vi "CSM - Check Status Registration.vi"(8 "error in (no error)":errorcluster, 10 "CSM Name":string, 11 "Broadcast state":string) -> (0 "error out":errorcluster, 3 "Array":T2(array[cluster]))   [LabVIEW 2017, in "Communicable State Machine.lvlib"]
doc: "-- <b>输入控件</b> --\n- <b>CSM Name</b>:\n- <b>Broadcast state</b>:\n\n-- <b>输出控件</b> --\n- <b>Array</b>:"
uses:
  Communicable State Machine.lvlib
  CSM - Broadcast Message Type.ctl
  Utility/Trim Both Whitespace.vi
  _Support/FGV-BroadcastRegistry/FGV-BroadcastRegistry.vi
  _Support/CSMQ/_CSMOFGV.vi
  _Support/BroadcastRegistry/HelperVI/Broadcast Item Key.vi
  _Support/FGV-BroadcastRegistry/global-Broadcast Cache Change Flag.vi
  _Support/FGV-BroadcastRegistry/global-CSMQ FGV Change Flag.vi
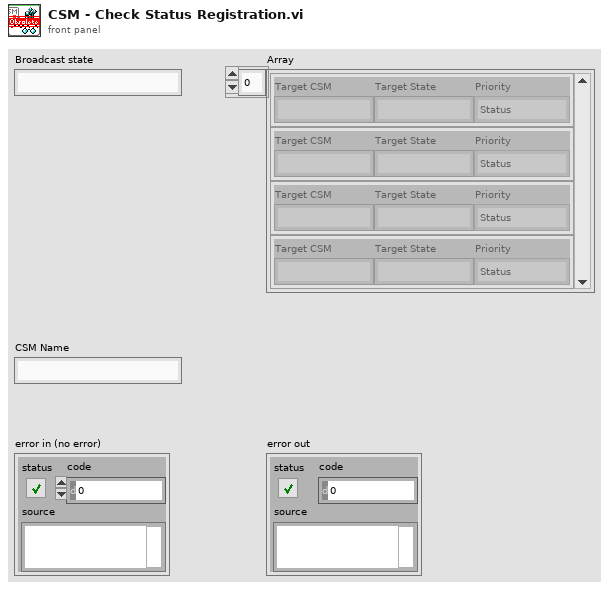
[diagram p1: front panel]
types:
  T1 = typedef "Communicable State Machine.lvlib/CSM - Broadcast Message Type.ctl" = enum16{"Status", "Interrupt(High)"}
  T2 = cluster{"Target CSM":string, "Target State":string, "Priority":T1}[]
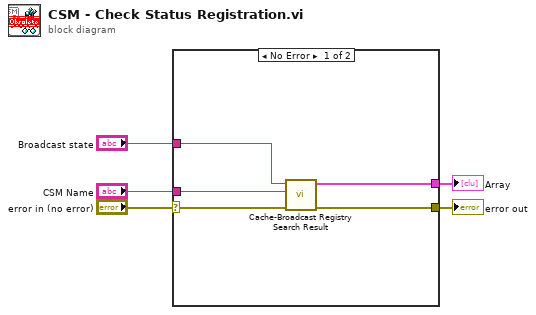
[diagram p0: block diagram]
diagram:
  n1 = case shown="No Error" "error in (no error)" {
    selector: "error in (no error)" -> [w7 w11]
    tunnel: "Broadcast state" -> [w10 _]
    tunnel: "CSM Name" -> [w9 _]
    tunnel: [w8 _] -> w3
    tunnel: [w6 w11] -> w1
    frame No Error {
      n2 = call "Cache-Broadcast Registry Search Result.vi"("error in (no error)"=w7, "CSM Name"=w9, "Broadcast state"=w10) -> ("error out"=w6:errorcluster, "Array"=w8:T2)  [unwired: 7 in]
    }
    frame Error {
    }
  }
  "Array" <- w3
  "error out" <- w1
